vi "Construct Flash Programming Command.vi"(7 "Flash Programming Command Type":T1, 8 "error in (no error)":errorcluster, 10 "Input":string) -> (0 "error out":errorcluster, 2 "Output":string)   [LabVIEW 2016, in "JLink Commander.lvlib"]
doc: "This VI constructs one target (CPU) configuration command string."
uses:
  JLink Commander.lvlib
  Type Definitions/Flash Programming Command Type Tab.ctl
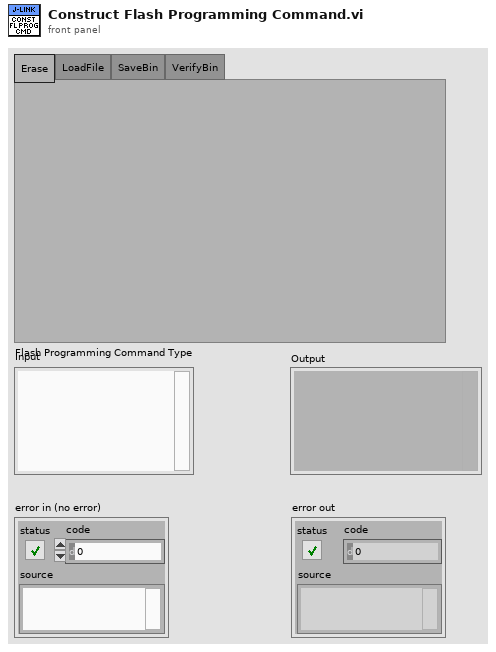
[diagram p1: front panel]
types:
  T1 = typedef "Flash Programming Command Type Tab.ctl" = enum32{"Erase", "LoadFile", "SaveBin", "VerifyBin"}
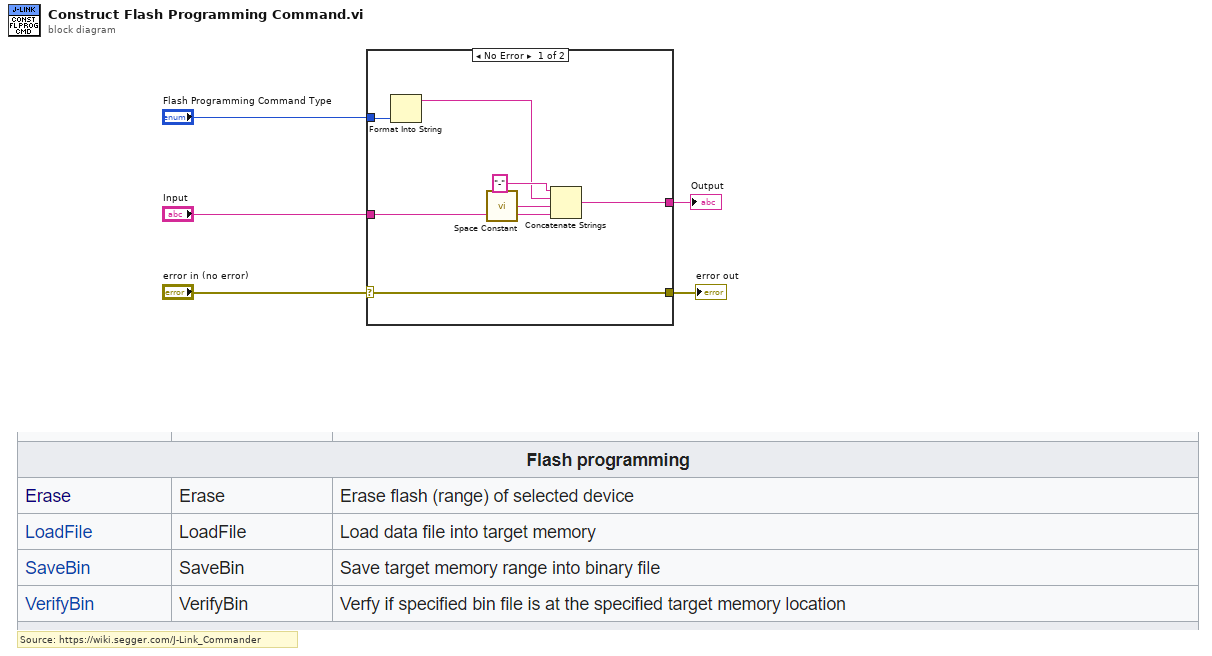
[diagram p0: block diagram]
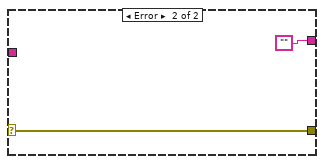
[diagram p2: hidden frame]
diagram:
  # "Source: https://wiki.segger.com/J-Link_Commander"
  n1 = case shown="No Error" "error in (no error)" {
    selector: "error in (no error)" -> [w8 w14]
    tunnel: [w8 w14] -> w5
    tunnel: [w12 ""] -> w4
    tunnel: "Input" -> [w9 _]
    tunnel: "Flash Programming Command Type" -> [w7 _]
    frame No Error {
      n2 = Format Into String(w7) -> (resulting string=w6:string)  [unwired: 3 in, 1 out]
      n3 = call <vilib>:"Space Constant.vi"() -> ("String"=w10:string)
      n4 = Concatenate Strings("-" ("string"), w6, w10, w9) -> (w12:string)
    }
    frame Error {
    }
  }
  "error out" <- w5
  "Output" <- w4
